vi "Hausmodell.WriteZustandsgrössen.vi"(0 "Hausmodell in":refnum<data-value>, 1 "Raumtemperatur [°C]":dbl, 2 "Bodentemperatur [°C]":dbl, 3 "Rücklauftemperatur Heizkreislauf [°C]":dbl, 5 "Error in":errorcluster) -> (19 "Error out":errorcluster)   [LabVIEW 2016, in "Hausmodell.lvclass"]
uses:
  Hausmodell.lvclass
  Hausmodell.lvclass/Hausmodell.ctl
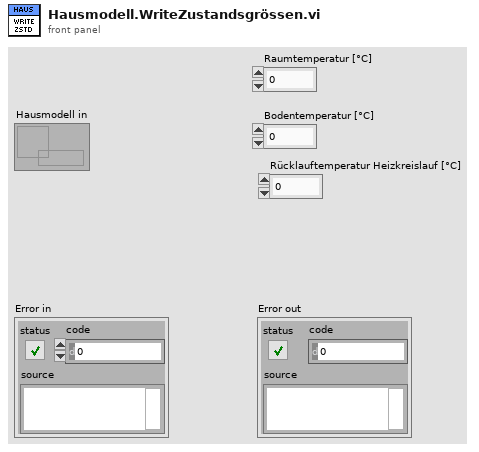
[diagram p1: front panel]
types:
  T1 = cluster{"Bodentemperatur [°C]":dbl, "Raumtemperatur [°C]":dbl, "Rücklauftemperatur Heizkreislauf [°C]":dbl}
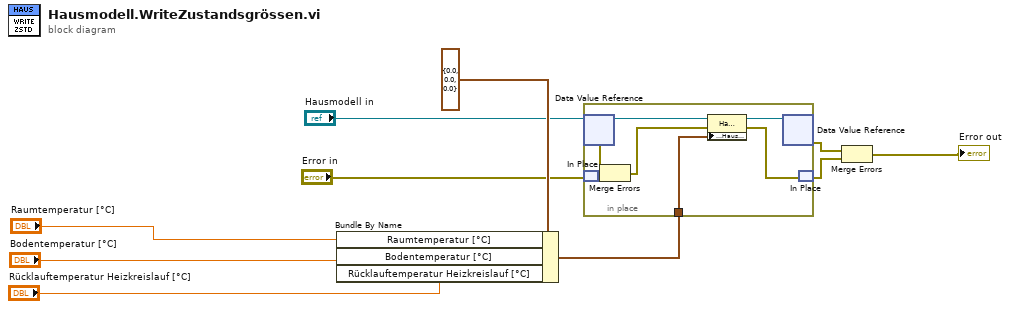
[diagram p0: block diagram]
diagram:
  n1 = Bundle By Name(cluster=T1 {"Bodentemperatur [°C]"=0.0, "Raumtemperatur [°C]"=0.0, "Rücklauftemperatur Heizkreislauf [°C]"=0.0} ("Zustandsgrössen.Hausmodell"), "Raumtemperatur [°C]"="Raumtemperatur [°C]", "Bodentemperatur [°C]"="Bodentemperatur [°C]", "Rücklauftemperatur Heizkreislauf [°C]"="Rücklauftemperatur Heizkreislauf [°C]") -> (w3:T1)
  n2 = in-place {
    in-place-border: w3 -> [w11]
    n3 = in-place-dvr #1("Hausmodell in") -> (w17:refnum<class "Hausmodell.lvclass">, w14:errorcluster)
    n4 = in-place-match #2("Error in") -> (w13:errorcluster)
    n5 = Merge Errors(w14, w13) -> (w15:errorcluster)
    n6 = property class="Hausmodell.lvclass"(reference=w17, error in=w15, "Accessors:Zustandsgrössen.Hausmodell"=w11) -> (reference out=w16:refnum<class "Hausmodell.lvclass">, error out=w12:errorcluster)
    n7 = in-place-dvr #1(w16) -> (w8:errorcluster)  [unwired: 1 out]
    n8 = in-place-match #2(w12) -> (w9:errorcluster)
  }
  n9 = Merge Errors(w8, w9) -> (→"Error out":errorcluster)
